vi "Picture.vi"(5 "Set Pictures (F)":bool, 7 "Pictures":picture[](array[picture]), 11 "Picture Item":T1) -> (3 "Picture":picture)   [LabVIEW 2020, in "VolatusGUIElements.lvlib" / "2WayValve.lvclass"]
uses:
  2WayValve.lvclass
  Picture.ctl
  2WayValve.lvclass/2WayValve.ctl
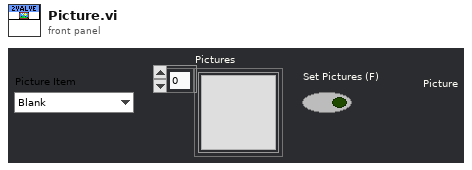
[diagram p1: front panel]
types:
  T1 = typedef "VolatusGUIElements.lvlib/2WayValve.lvclass/Picture.ctl" = enum16{"Blank", "OutClose", "OutOpen", "OutTranClose", "OutTranOpen", "OutConfig", "OutStale", "OutError", "InClose", "InOpen", "InTranClose", "InTranOpen", "InConfig", "InStale", "InError", "EnOff", "EnOn", "EnConfig", "EnStale", "EnError"}
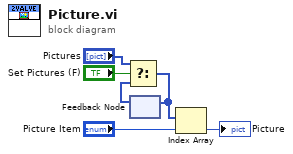
[diagram p0: block diagram]
diagram:
  n1 = feedback #1() -> (w3:picture[])  [unwired: 1 in]
  n2 = Select(t="Pictures", s="Set Pictures (F)", f=w3) -> (s? t:f=w2:picture[])
  n3 = feedback-in #1(w2) -> ()
  n4 = Index Array(array=w2, index="Picture Item") -> (element=→"Picture":picture)
